vi "HB_Society.appendData2Variant.vi"(0 "initData":variant, 2 "nofPersons":i32, 5 "error in (no error)":errorcluster) -> (14 "dup initData":variant, 19 "error out":errorcluster)   [LabVIEW 2009, in "HB_BaseClass_Examples.lvlib" / "HB_Society.lvclass"]
doc: "Append initialize data to variant."
uses:
  HB_Society.lvclass
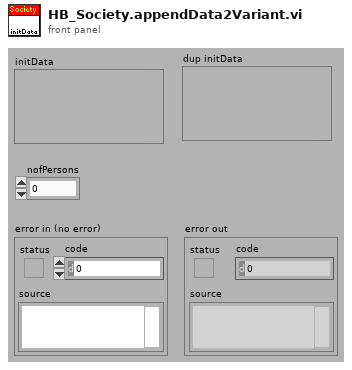
[diagram p1: front panel]
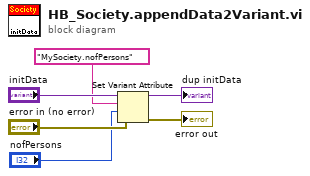
[diagram p0: block diagram]
diagram:
  n1 = Set Variant Attribute(Variant="initData", name="MySociety.nofPersons", value="nofPersons", error in="error in (no error)") -> (Variant out=→"dup initData":variant, error out=→"error out":errorcluster)  [unwired: 1 out]
